vi "숫자판.vi"() -> ()   [LabVIEW 2018]
uses:
  <vilib>/DAQmx/write.llb/DAQmx Write (Digital 1D Bool 1Chan 1Samp).vi
  <vilib>/DAQmx/create/channels.llb/DAQmx Create Channel (DO-Digital Output).vi
  <vilib>/DAQmx/miscellaneous.llb/DAQmx Fill In Error Info.vi
panel:
  in  "lines":tag caption="라인"
  out "클러스터":T1
  in  "정지 버튼":bool
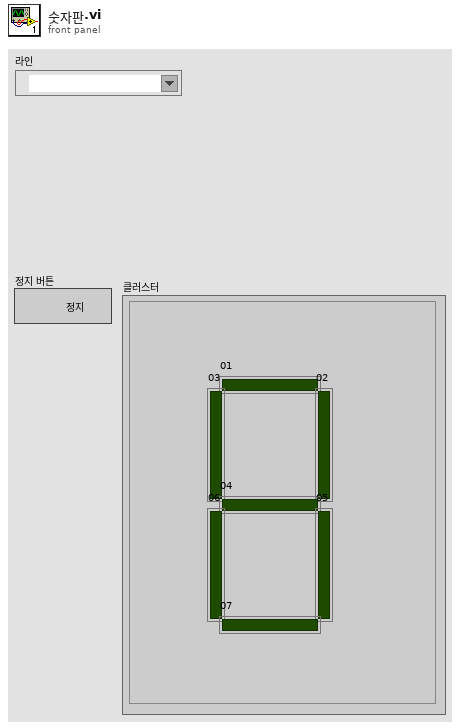
[diagram p1: front panel]
types:
  T1 = cluster{"01":bool, "02":bool, "03":bool, "04":bool, "05":bool, "06":bool, "07":bool}
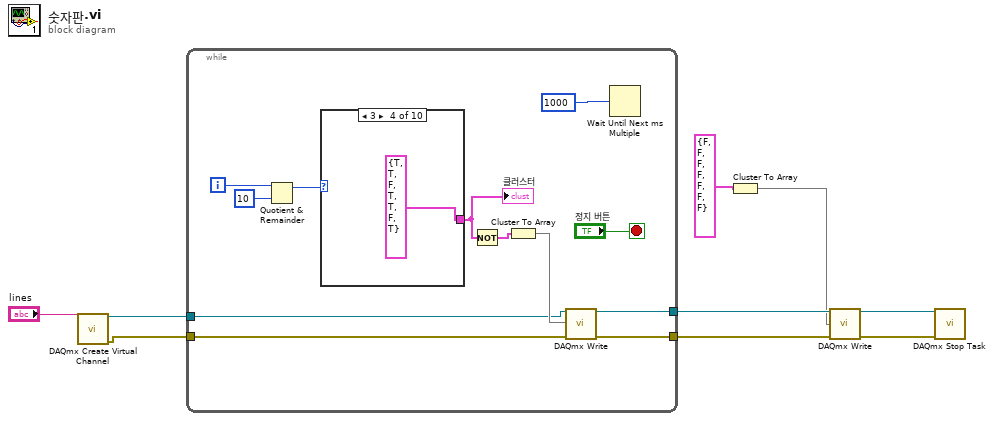
[diagram p0: block diagram]
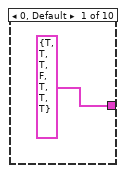
[diagram p2: hidden frame]
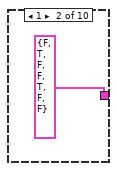
[diagram p3: hidden frame]
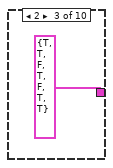
[diagram p4: hidden frame]
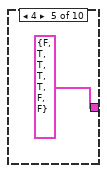
[diagram p5: hidden frame]
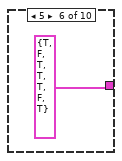
[diagram p6: hidden frame]
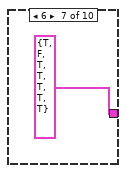
[diagram p7: hidden frame]
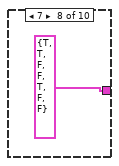
[diagram p8: hidden frame]
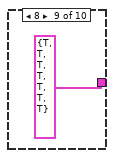
[diagram p9: hidden frame]
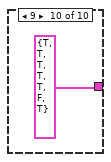
[diagram p10: hidden frame]
diagram:
  n1 = call-poly <vilib>:"DAQmx Create Virtual Channel.vi"("lines"="lines") -> ("task out"=w8:refnum<k21>, "error out"=w7:errorcluster)  [unwired: 13 in]
  n2 = while {
    tunnel: w8 -> [w13]
    tunnel: w7 -> [w12]
    tunnel: [w11] -> w6
    tunnel: [w10] -> w5
    i -> [w19]
    stop <- "정지 버튼" stop-if-true
    n3 = Quotient & Remainder(x=w19, y=10) -> (x-y*floor(x/y)=w17:i32)  [unwired: 1 out]
    n4 = case shown="3" w17 {
      tunnel: [T1 {"01"=TRUE, "02"=TRUE, "03"=TRUE, "04"=FALSE, "05"=TRUE, "06"=TRUE, "07"=TRUE} ("클러스터") T1 {"01"=FALSE, "02"=TRUE, "03"=FALSE, "04"=FALSE, "05"=TRUE, "06"=FALSE, "07"=FALSE} ("클러스터") T1 {"01"=TRUE, "02"=TRUE, "03"=FALSE, "04"=TRUE, "05"=FALSE, "06"=TRUE, "07"=TRUE} ("클러스터") T1 {"01"=TRUE, "02"=TRUE, "03"=FALSE, "04"=TRUE, "05"=TRUE, "06"=FALSE, "07"=TRUE} ("클러스터") T1 {"01"=FALSE, "02"=TRUE, "03"=TRUE, "04"=TRUE, "05"=TRUE, "06"=FALSE, "07"=FALSE} ("클러스터") T1 {"01"=TRUE, "02"=FALSE, "03"=TRUE, "04"=TRUE, "05"=TRUE, "06"=FALSE, "07"=TRUE} ("클러스터") T1 {"01"=TRUE, "02"=FALSE, "03"=TRUE, "04"=TRUE, "05"=TRUE, "06"=TRUE, "07"=TRUE} ("클러스터") T1 {"01"=TRUE, "02"=TRUE, "03"=FALSE, "04"=FALSE, "05"=TRUE, "06"=FALSE, "07"=FALSE} ("클러스터") T1 {"01"=TRUE, "02"=TRUE, "03"=TRUE, "04"=TRUE, "05"=TRUE, "06"=TRUE, "07"=TRUE} ("클러스터") T1 {"01"=TRUE, "02"=TRUE, "03"=TRUE, "04"=TRUE, "05"=TRUE, "06"=FALSE, "07"=TRUE} ("클러스터")] -> w16
      frame 0, Default {
      }
      frame 1 {
      }
      frame 2 {
      }
      frame 3 {
      }
      frame 4 {
      }
      frame 5 {
      }
      frame 6 {
      }
      frame 7 {
      }
      frame 8 {
      }
      frame 9 {
      }
    }
    "클러스터" <- w16
    n5 = Not(x=w16) -> (.not. x?=w15:T1)
    n6 = Cluster To Array(cluster=w15) -> (array=w14:bool[])
    n7 = call-poly <vilib>:"DAQmx Write.vi"("task/channels in"=w13, "data"=w14, "error in"=w12) -> ("task out"=w11:refnum<k21>, "error out"=w10:errorcluster)  [unwired: 10 in, 1 out]
    n8 = Wait Until Next ms Multiple(millisecond multiple=u32 1000 ("ms 배수")) -> ()  [unwired: 1 out]
  }
  n9 = Cluster To Array(cluster=T1 {"01"=FALSE, "02"=FALSE, "03"=FALSE, "04"=FALSE, "05"=FALSE, "06"=FALSE, "07"=FALSE} ("클러스터")) -> (array=w3:bool[])
  n10 = call-poly <vilib>:"DAQmx Write.vi"("task/channels in"=w6, "data"=w3, "error in"=w5) -> ("task out"=w2:refnum<k21>, "error out"=w1:errorcluster)  [unwired: 10 in, 1 out]
  n11 = call <vilib>:"DAQmx Stop Task.vi"("task/channels in"=w2, "error in"=w1) -> ()  [unwired: 12 in, 2 out]
